vi "Pre Launch Init.vi"(11 "[V]System Tree View in":refnum<class "[V]System Tree View.lvclass">) -> (0 "error out":errorcluster, 3 "[V]System Tree View out":refnum<class "[V]System Tree View.lvclass">)   [LabVIEW 2020, in "[V]System Tree View.lvlib" / "[V]System Tree View.lvclass"]
doc: "(<B>Filename</B>: Actor Framework.lvlib:Actor.lvclass:Pre Launch Init.vi)\n\nDefines behavior that occurs after the Launch Nested Actor method is invoked but before the actor's Actor Core method begins running.\n\nBy default, this method does nothing. A descendant class may override it to define behavior."
uses:
  [V]System Tree View.lvclass
  Depden On/MVVM Framework/MVVM Abstruct View/MVVM Abstruct View/MVVM Abstruct View.lvclass
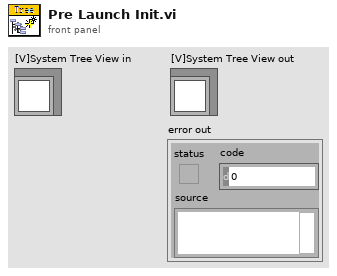
[diagram p1: front panel]
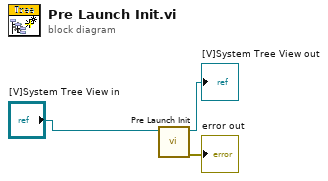
[diagram p0: block diagram]
diagram:
  n1 = call-parent "Pre Launch Init.vi"("Abstruct View in"="[V]System Tree View in") -> ("error out"=→"error out":errorcluster, "Abstruct View out"=→"[V]System Tree View out":refnum<class "[V]System Tree View.lvclass">)  [unwired: 9 in]
